vi "PH_gentec_P-Link.destructor.vi"(0 "i ref in":refnum<vi>, 5 "error in(no error)":errorcluster) -> (19 "error out":errorcluster)   [LabVIEW 2014, in "PH_gentec_P-Link.lvlib"]
doc: "This is the destructor of a class.\n\nLicense Agreement for this software:\n\nCopyright (C)\nGesellschaft für Schwerionenforschung, GSI\nPlanckstr. 1\n64291 Darmstadt\nGermany\n\nContact: D.Beck@gsi.de \n\nThis program is free software; you can redistribute it and/or modify it under the terms of the \nGNU General Public License as published by the Free Software Foundation; either version 2 of \nthe license, or (at your option) any later version.\n\nThis program is distributed in the hope that it will be useful, but WITHOUT ANY WARRANTY; \nwithout even the implied warranty of MERCHANTABILITY or FITNESS FOR A PARTICULAR PURPOSE. See the GNU General License for more details (http://www.gnu.org).\n\nGesellschaft für Schwerionenforschung, GSI\nPlanckstr. 1, 64291 Darmstadt, Germany\nFor all questions and ideas contact: M.Richter@gsi.de, H.Brand@gsi.de or D.Beck@gsi.de.\nLast update: 16-JUN-2004"
uses:
  PH_gentec_P-Link.lvlib
  PH_Basics/PH_Powermeter_BaseClass/PH_Powermeter_BaseClass.State.ctl
  instr.lib/Gentec-M-Link/gentec-M-Link - Driver.lvlib
  PH_Basics/PH_Powermeter_BaseClass/PH_Powermeter_BaseClass.lvlib
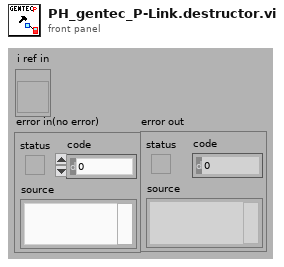
[diagram p1: front panel]
types:
  T1 = typedef "PH_Powermeter_BaseClass.lvlib/PH_Powermeter_BaseClass.State.ctl" = enum32{"off", "operating", "opened", "checked", "connected", "Sets to change", "running"}
  T2 = typedef "PH_Powermeter_BaseClass.lvlib/PH_Powermeter_BaseClass.i attribute.ctl" = cluster{"GUI References":T3, "Connection":T4, "Head Attributes":T5, "VISA resource":refnum<visa-resource-name>, "Energy":T6, "Service ID Energy":i32, "Wanted Settings":T7, "Current Settings":T7}
  T3 = typedef "PH_Powermeter_BaseClass.lvlib/PH_Powermeter_BaseClass.GUI Refs.ctl" = cluster{"Head Attributes":refnum<vi>, "Energy":refnum<vi>, "Connection":refnum<vi>, "VISA Resource":refnum<vi>, "Scaling Factor":refnum<vi>, "Range":refnum<vi>, "Wavelength":refnum<vi>, "Trigger Level":refnum<vi>, "Wanted Settings":refnum<vi>, "Current Settings":refnum<vi>}
  T4 = typedef "PH_Powermeter_BaseClass.lvlib/PH_Powermeter_BaseClass.Connection.ctl" = cluster{"failed checks":i8, "Timeout":bool, "Data read":string, "Failure":bool, "Error":bool, "State":T1}
  T5 = typedef "PH_Powermeter_BaseClass.lvlib/PH_Powermeter_BaseClass.Head Attributes.ctl" = cluster{"Instrument Type":string, "Head Version":string, "Head Name":string, "Serial Number":string, "Firmware":string, "Sensor Type":string, "MinimumRange":u32, "Maximum Range":u32, "Min Wavelength":i32, "Max Wavelength":i32}
  T6 = typedef "PH_Powermeter_BaseClass.lvlib/PH_Powermeter_BaseClass.Energy.ctl" = cluster{"current Value":dbl, "unscaled":dbl, "Scaling Factor":dbl}
  T7 = typedef "PH_Powermeter_BaseClass.lvlib/PH_gentec_BaseClass.Head Settings.ctl" = cluster{"Trigger Level":dbl, "Wavelength":u32, "Range":u32}
  T8 = typedef "PH_gentec_P-Link.lvlib/PH_gentec_P-Link.i attribute.ctl" = cluster{"GUI References":cluster{"Wanted Head Settings":refnum<vi>, "Current Head Settings":refnum<vi>, "Set Auto Range":refnum<vi>, "Trigger Polarity":refnum<vi>, "Trigger Source":refnum<vi>, "Waveform Averages":refnum<vi>, "Continuous":refnum<vi>, "get one Value":refnum<vi>, "Set Zero":refnum<vi>}, "Wanted Head Settings":T9, "Current Head Settings":T9}
  T9 = typedef "PH_gentec_P-Link.lvlib/PH_gentec_P-Link.Head Settings.ctl" = cluster{"Enable Anticipation":bool, "Set Auto Range":bool, "Set Zero":i32, "Current":i32, "Start Data Flow":bool}
  T10 = enum16{"SetAttribute", "GetAttribute", "CreateAttribute", "DestroyAttribute", "DestroyAllAtributes"}
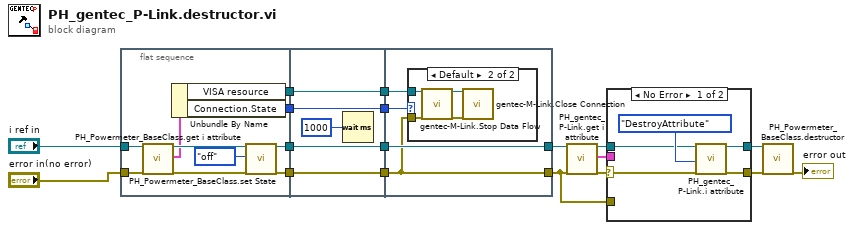
[diagram p0: block diagram]
diagram:
  n1 = flat-sequence {
    tunnel: "error in(no error)" -> [w25]
    tunnel: "i ref in" -> [w24]
    tunnel: [w27] -> w14
    tunnel: [w28] -> w13
    tunnel: [w20] -> w4
    tunnel: [w19] -> w1
    tunnel: w14 -> [w33]
    tunnel: w13 -> [w32]
    tunnel: [w33] -> w6
    tunnel: [w32] -> w5
    tunnel: w4 -> [w30]
    tunnel: [w30] -> w3
    tunnel: [w29] -> w2
    tunnel: w1 -> [w29]
    tunnel: [w35] -> w8
    tunnel: [w34] -> w7
    tunnel: w6 -> [w34]
    tunnel: w5 -> [w35]
    tunnel: w3 -> [w37]
    tunnel: w2 -> [w36]
    frame #0 {
      n2 = call "PH_Powermeter_BaseClass.get i attribute.vi"("i ref in"=w24, "error in (no error)"=w25) -> ("i ref out"=w22:refnum<vi>, "i attribute"=w21:T2, "error out"=w23:errorcluster)  [unwired: 15 in]
      n3 = Unbundle By Name(w21) -> ("VISA resource"=w20:refnum<visa-resource-name>, "Connection.State"=w19:T1)
      n4 = call "PH_Powermeter_BaseClass.set State.vi"("VI in"=w22, "State"=PH_Powermeter_BaseClass.State."off", "error in (no error)"=w23) -> ("VI out"=w28:refnum<vi>, "error out"=w27:errorcluster)  [unwired: 15 in]
    }
    frame #1 {
      n5 = Wait (ms)(milliseconds to wait=u32 1000) -> ()  [unwired: 1 out]
    }
    frame #2 {
      n6 = case shown="Default" w36 {
        tunnel: w34 -> [_ w41]
        tunnel: w37 -> [_ w39]
        frame "off", "operating" {
        }
        frame Default {
          n7 = call "gentec-M-Link.Stop Data Flow.vi"("VISA resource In"=w39, "error in (no error)"=w41) -> ("VISA resource Out"=w38:refnum<visa-resource-name>, "error out"=w40:errorcluster)  [unwired: 13 in, 3 out]
          n8 = call "gentec-M-Link.Close Connection.vi"("VISA resource In"=w38, "error in (no error)"=w40) -> ()  [unwired: 17 in, 1 out]
        }
      }
    }
  }
  n9 = call "PH_gentec_P-Link.get i attribute.vi"("i ref in"=w8, "error in (no error)"=w7) -> ("i ref out"=w12:refnum<vi>, "i attribute"=w17:T8, "error out"=w10:errorcluster)  [unwired: 15 in]
  n10 = case shown="No Error" w10 {
    selector: w10 -> [w42 _]
    tunnel: [w45 w48] -> w18
    tunnel: w17 -> [_ _]
    tunnel: w12 -> [w44 w47]
    tunnel: [w43 w47] -> w11
    tunnel: w7 -> [_ w48]
    frame No Error {
      n11 = call "PH_gentec_P-Link.i attribute.vi"("VI Refnum"=w44, "Action"=T10."DestroyAttribute", "error in (no error)"=w42) -> ("VI Refnum out"=w43:refnum<vi>, "error out"=w45:errorcluster)  [unwired: 14 in, 1 out]
    }
    frame Error {
    }
  }
  n12 = call "PH_Powermeter_BaseClass.destructor.vi"("i ref in"=w11, "error in(no error)"=w18) -> ("error out"=→"error out":errorcluster)  [unwired: 17 in]
